vi "E709_Sample_Application_With_Analog.vi"() -> ()   [LabVIEW 2014, in "PiFOC.lvlib"]
doc: "This VI demonstrates the use of digital (e.g. RS-232) communication and analog interfacing in parallel for the E-709. \n\nIn this example the E-709 is connected through COM port 1 with baudrate 57600. The VI first initializes the E-709 via the selected digital interface by running \"E709_Configuration_Setup.vi\". It then switches to analog control, using \"SwitchToAnalogOrDigital.vi\" and initializes the analog interface by running \"Analog_Configuration_Setup.vi\". After these initialization steps, it moves one axis relative to its current position by outputting a voltage by the DAC card used, waits 10 ms and queries for the position of this axis. Finally, it switches back to digital control and closes both the analog and the digital connection to the controller. \nThe diagram shows how to combine the driver VIs for these tasks. \nWarning: Before running this VI, modify the \"Interface\" and \"RS232 settings\" (or \"USB settings\") to reflect your configuration. The predefined settings provided with the VI probably do not match your system.\nBoth the E-709 Digital LabVIEW driver set and the GCS Analog LabVIEW driver set must be installed, otherwise the VI will not be executable."
uses:
  PiFOC.lvlib
panel:
  out "Running 2":bool caption="Analog_Configuration_Setup.vi is running"
  in  "stop":bool
  in  "error in":errorcluster
  out "Running":bool caption="E709_Configuration_Setup.vi is running"
  out "error out":errorcluster
  out "Position":dbl[](array[numeric]) format="%.6f"
  out "Conn. Axis":string[](array[string])
  out "E-709 Identification":string
  # "This This VI demonstrates the use of digital (e.g. RS-232) communication and analog interfacing in parallel for the E-709.  The diagram\nshows how to combine the driver VIs for these tasks.\n\nWarning: Before running this VI, modify the interface settings on the block diagram to reflect your configuration. The predefined \n                 settings provided with the VI probably do not match your system.\n                 Both the E-709 Digital LabVIEW driver set and the GCS Analog LabVIEW driver set must be installed, otherwise the VI will not\n                 be executable."
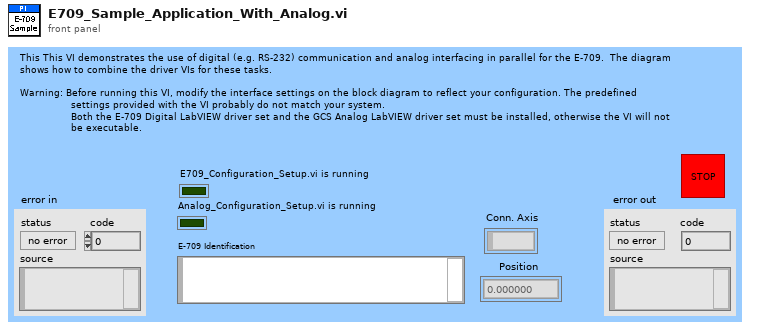
[diagram p1: front panel]
types:
  T1 = cluster{"Conn. Axes":string[], "AI channels":tag[], "AO channels":tag[], "Lower voltage limit (V)":dbl, "Upper voltage limit (V)":dbl, "AI Sample Rate":dbl, "AI Samples/Channel":i32}
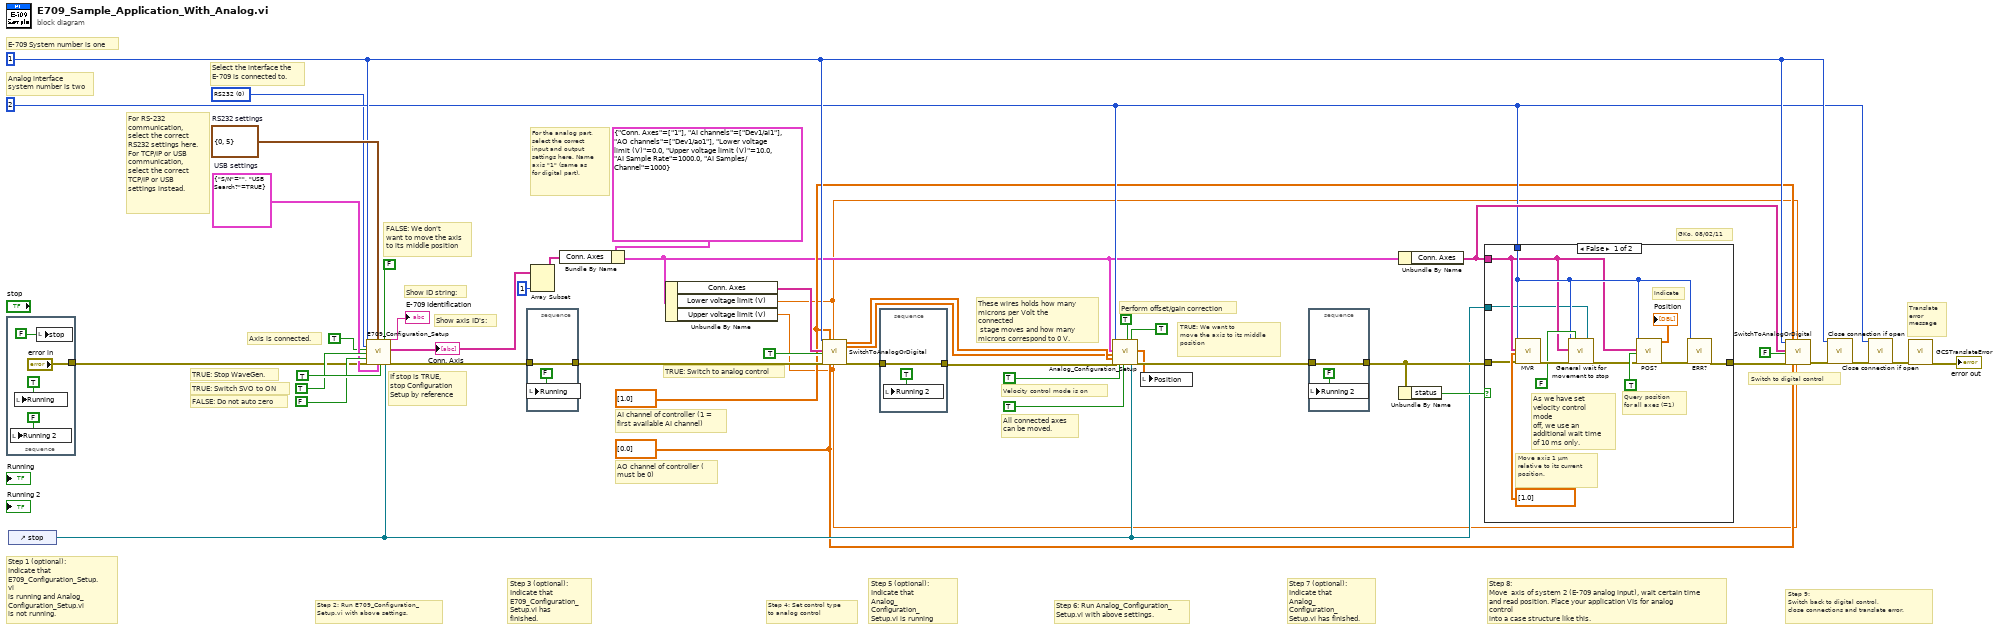
[diagram p0: block diagram]
diagram:
  w1 = u16 0 items=["RS232", "USB", "RS232 DaisyChain"] ("Interface")
  w11 = dbl[] [0.0] ("AO channels")
  w12 = dbl[] [1.0] ("AI channels")
  w14 = 2 ("System no.")
  w32 = cluster{"S/N":string, "USB Search?":bool} {"S/N"="", "USB Search?"=TRUE}  # USB settings
  w38 = cluster{"Portnumber":i32, "Baudrate":u16} {"Portnumber"=0, "Baudrate"=5}  # RS232 settings
  w15 = 1 ("System no.")
  # "GKo, 08/02/11"
  # "Step 7 (optional):\nIndicate that\nAnalog_Configuration_\nSetup.vi has finished."
  # "Step 5 (optional):\nIndicate that\nAnalog_Configuration_\nSetup.vi is running"
  # "Step 3 (optional):\nIndicate that\nE709_Configuration_\nSetup.vi has finished."
  # "Step 4: Set control type\nto analog control"
  # "Step 9: \nSwitch back to digital control,\nclose connections and translate error."
  # "Translate\nerror \nmessage"
  # "Switch to digital control"
  # "AO channel of controller (\nmust be 0)"
  # "AI channel of controller (1 = \nfirst available AI channel)"
  # "TRUE: Switch to analog control"
  # "Step 6: Run Analog_Configuration_\nSetup.vi with above settings."
  # "Velocity control mode is on"
  # "TRUE: We want to\nmove the axis to its middle\nposition"
  # "Perform offset/gain correction"
  # "All connected axes\ncan be moved."
  # "These wires holds how many\nmicrons per Volt the connected\n stage moves and how many\nmicrons correspond to 0 V."
  # "For the analog part,\nselect the correct\ninput and output \nsettings here. Name\naxis \"1\" (same as \nfor digital part)."
  # "Analog interface \nsystem number is two"
  # "Axis is connected."
  # "FALSE: We don't\nwant to move the axis\nto its middle position"
  # "FALSE: Do not auto zero"
  # "TRUE: Switch SVO to ON"
  # "If stop is TRUE, \nstop Configuration\nSetup by reference"
  # "Step 8: \nMove  axis of system 2 (E-709 analog input), wait certain time\nand read position. Place your application VIs for analog control\ninto a case structure like this."
  # "For RS-232 \ncommunication,\nselect the correct\nRS232 settings here.\nFor TCP/IP or USB \ncommunication, \nselect the correct \nTCP/IP or USB\nsettings instead."
  # "Select the interface the \nE-709 is connected to."
  # "Step 2: Run E709_Configuration_\nSetup.vi with above settings."
  # "Step 1 (optional): \nIndicate that\nE709_Configuration_Setup.vi\nis running and Analog_\nConfiguration_Setup.vi\nis not running."
  # "Show axis ID's:"
  # "Show ID string:"
  # "TRUE: Stop WaveGen."
  # "E-709 System number is one"
  n1 = stacked-sequence {
    tunnel: ["error in"] -> w23
    frame #0 {
      n2 = local write "Running 2"(FALSE ("Running")) -> ()
      n3 = local write "Running"(TRUE ("Running")) -> ()
      n4 = local write "stop"(FALSE ("stop")) -> ()
    }
  }
  n5 = control-ref of="stop"() -> (w24:refnum<vi>)
  n6 = call "E709_Configuration_Setup.vi"("System no."=w15, "Interface"=w1, "Connected?"=TRUE, "Change servo status to ON?"=TRUE ("Use dialog to define\nconnected stages?"), "Perform autozero?"=FALSE ("Use dialog to define\nconnected stages?"), "error in"=w23, "RS232 settings"=w38, "USB settings"=w32, "Stop wave generator\noutput (if any)"=TRUE ("All axes?"), "Move to middle?"=FALSE, "Stop refnum"=w24) -> ("Identification"=→"E-709 Identification":string, "Conn. \nAxis"=w3:string[], "error out"=w19:errorcluster)  [unwired: 3 in, 3 out]
  "Conn. Axis" <- w3
  n7 = stacked-sequence {
    tunnel: w19 -> [w51]
    tunnel: [w51] -> w20
    frame #0 {
      n8 = local write "Running"(FALSE ("Running")) -> ()
    }
  }
  n9 = Array Subset(array=w3, length=1) -> (w2:string[])  [unwired: 1 in]
  n10 = Bundle By Name(cluster=T1 {"Conn. Axes"=["1"], "AI channels"=["Dev1/ai1"], "AO channels"=["Dev1/ao1"], "Lower voltage limit (V)"=0.0, "Upper voltage limit (V)"=10.0, "AI Sample Rate"=1000.0, "AI Samples/Channel"=1000} ("Input/output settings"), "Conn. Axes"=w2) -> (w8:T1)
  n11 = Unbundle By Name(w8) -> ("Conn. Axes"=w26:string[], "Lower voltage limit (V)"=w7:dbl, "Upper voltage limit (V)"=w6:dbl)
  n12 = call "SwitchToAnalogOrDigital.vi"("System no."=w15, "Axes to command"=w26, "Mode"=TRUE ("Mode (Analog: T)"), "error in"=w20, "AI channels"=w12, "AO channels"=w11, "Lower voltage limit (V)"=w7, "Upper voltage limit (V)"=w6) -> ("Conversion factor"=w30:dbl[], "Offset"=w13:dbl[], "Error out"=w22:errorcluster)  [unwired: 3 in, 6 out]
  n13 = stacked-sequence {
    tunnel: [w52] -> w21
    tunnel: w22 -> [w52]
    frame #0 {
      n14 = local write "Running 2"(TRUE ("Running")) -> ()
    }
  }
  n15 = call "Analog_Configuration_Setup.vi"("System no."=w14, "Input/output settings"=w8, "Conversion offset"=w13, "Conversion factor"=w30, "error in"=w21, "Vel. control mode"=TRUE, "All axes?"=TRUE, "Offset/Gain\ncorrection"=TRUE ("Offset/Gain\ncorrection"), "Move \nto middle?"=TRUE ("Move \nto middle?"), "Stop refnum"=w24) -> ("Position"=w5:dbl[], "error out"=w37:errorcluster)  [unwired: 3 in, 5 out]
  n16 = local write "Position"(w5) -> ()
  n17 = stacked-sequence {
    tunnel: w37 -> [w55]
    tunnel: [w55] -> w44
    frame #0 {
      n18 = local write "Running 2"(FALSE ("Running")) -> ()
    }
  }
  n19 = Unbundle By Name(w8) -> ("Conn. Axes"=w25:string[])
  n20 = Unbundle By Name(w44) -> ("status"=w43:bool)
  n21 = case shown="False" w43 {
    tunnel: [w56 w68] -> w27
    tunnel: w44 -> [w59 w68]
    tunnel: w24 -> [w57 _]
    tunnel: w14 -> [w61 _]
    tunnel: w25 -> [w58 _]
    frame False {
      # "As we have set\nvelocity control mode\noff, we use an\nadditional wait time\nof 10 ms only."
      # "Indicate"
      # "Query position\nfor all axes (=1)"
      # "Move axis 1 µm\nrelative to its current\nposition."
      n22 = call "MVR.vi"("System no."=w61, "Axes to move"=w58, "Position values"=dbl[] [1.0], "error in"=w59) -> ("error out"=w65:errorcluster)  [unwired: 1 in, 14 out]
      n23 = call "General wait for movement to stop.vi"("System no."=w61, "Axes to wait for"=w58, "error in"=w65, "Add. wait only?"=FALSE, "Stop refnum"=w57) -> ("error out"=w64:errorcluster)  [unwired: 3 in, 11 out]
      n24 = call "POS?.vi"("System no."=w61, "Axes to query"=w58, "All axes?"=TRUE, "error in"=w64) -> ("Position"=→"Position":dbl[], "error out"=w63:errorcluster)  [unwired: 1 in, 13 out]
      n25 = call "ERR?.vi"("System no."=w61, "error in"=w63) -> ("error out"=w56:errorcluster)  [unwired: 17 out]
    }
    frame True {
      # "Error during initialization"
    }
  }
  n26 = call "SwitchToAnalogOrDigital.vi"("System no."=w15, "Axes to command"=w25, "Mode"=FALSE, "error in"=w27, "AI channels"=w12, "AO channels"=w11, "Lower voltage limit (V)"=w7, "Upper voltage limit (V)"=w6) -> ("Error out"=w18:errorcluster)  [unwired: 1 in, 10 out]
  n27 = call "Close connection if open.vi"("System no."=w15, "error in"=w18) -> ("error out"=w17:errorcluster)  [unwired: 1 in, 16 out]
  n28 = call "Close connection if open.vi"("System no."=w14, "error in"=w17) -> ("error out"=w16:errorcluster)  [unwired: 1 in, 16 out]
  n29 = call "GCSTranslateError.vi"("error in"=w16) -> ("error out"=→"error out":errorcluster)  [unwired: 18 out]
